vi "test_Generate State Information (JSON RCT).vi"(8 "error in":errorcluster) -> (0 "error out":errorcluster)   [LabVIEW 2020, in "Test_Routing Templates.lvlib"]
uses:
  Test_Routing Templates.lvlib
  Shared/Routing State.ctl
  Shared/Connection.ctl
  Routing Channel Templates/Abstract Routing Channel Template/Abstract Routing Channel Template.lvclass/Abstract Routing Channel Template.ctl
  Routing Channel Templates/JSON Routing Channel Template/JSON Routing Channel Template.lvclass
  C:/Users/mjacobso/Desktop/SCM/Routing-Faulting/Source/Routing and Faulting/Routing Templates/Routing Channel Templates/Abstract Routing Channel Template/Abstract Routing Channel Template.lvclass
  <vilib>/addons/_JKI Toolkits/Caraya/classes/Assert/Assert Equal Value_Variant.vi
  <vilib>/addons/_JKI Toolkits/Caraya/classes/Assert/Assert Error.vi
  <vilib>/addons/_JKI Toolkits/Caraya/classes/Test/Test.lvclass
  <vilib>/addons/_JKI Toolkits/Caraya/classes/Assert/Assert.lvclass
  Routing Channel Templates/Abstract Routing Channel Template/Abstract Routing Channel Template.lvclass
  Shared/Routing and Faulting Shared.lvlib
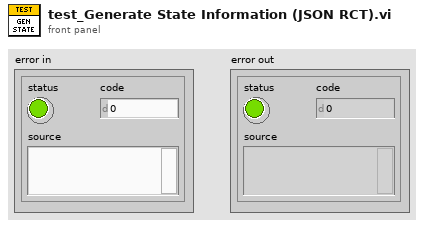
[diagram p1: front panel]
types:
  T1 = typedef "Routing and Faulting Shared.lvlib/Routing State.ctl" = cluster{"Name":string, "Description":string, "Value":i32, "Connection List":T2[]}
  T2 = typedef "Routing and Faulting Shared.lvlib/Connection.ctl" = cluster{"Module":string, "Source":string, "Destination":string}
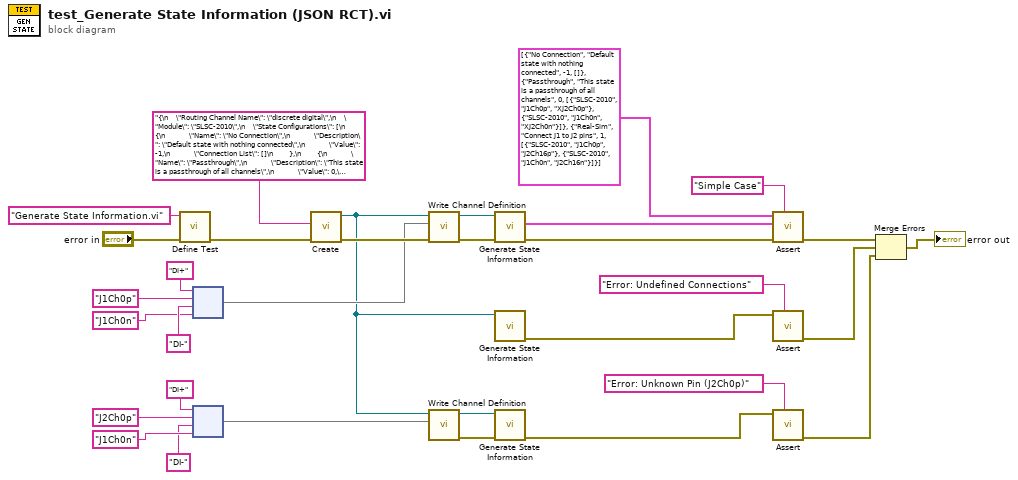
[diagram p0: block diagram]
diagram:
  n1 = call <vilib>:"Define Test.vi"("error in (no error)"="error in", "Label (VI Title)"="Generate State Information.vi") -> ("error out"=w29:errorcluster)  [unwired: 9 in]
  n2 = node("DI+", "J1Ch0p", "DI-", "J1Ch0n") -> (w22:map{string, string})
  n3 = node("DI+", "J2Ch0p", "DI-", "J1Ch0n") -> (w1:map{string, string})
  n4 = call "Create.vi"("error in (no error)"=w29, "JSON"="{\n    \"Routing Channel Name\": \"discrete digital\",\n    \"Module\": \"SLSC-2010\",\n    \"State Configurations\": [\n        {\n            \"Name\": \"No Connection\",\n            \"Description\": \"Default state with nothing connected\",\n            \"Value\": -1,\n            \"Connection List\": []\n        },\n        {\n            \"Name\": \"Passthrough\",\n            \"Description\": \"This state is a passthrough of all channels\",\n            \"Value\": 0,\n            \"Connection List\": [\n                {\n                    \"Channel\": \"DI+\",\n                    \"Connection Type\": \"Passthrough\"\n                },\n                {\n                    \"Channel\": \"DI-\",\n                    \"Connection Type\": \"Passthrough\"\n                }\n            ]\n        },\n        {\n            \"Name\": \"Real-Sim\",\n            \"Description\": \"Connect J1 to J2 pins\",\n            \"Value\": 1,\n            \"Connection List\": [\n                {\n                    \"Channel\": \"DI+\",\n                    \"Connection Type\": \"Real-Sim\"\n                },\n                {\n                    \"Channel\": \"DI-\",\n                    \"Connection Type\": \"Real-Sim\"\n                }\n            ]\n        }\n    ]\n}" ("text")) -> ("error out"=w27:errorcluster, "JSON Routing Channel Template out"=w8:refnum<class "JSON Routing Channel Template.lvclass">)  [unwired: 8 in]
  n5 = call "Write Channel Definition.vi"("error in (no error)"=w27, "Channel Definition"=w22, "Abstract Routing Channel Template in"=w8) -> ("error out"=w20:errorcluster, "Abstract Routing Channel Template out"=w19:refnum<class "JSON Routing Channel Template.lvclass">)  [unwired: 7 in]
  n6 = call "Write Channel Definition.vi"("Channel Definition"=w1, "Abstract Routing Channel Template in"=w8) -> ("error out"=w10:errorcluster, "Abstract Routing Channel Template out"=w9:refnum<class "JSON Routing Channel Template.lvclass">)  [unwired: 8 in]
  n7 = call-dynamic "Generate State Information.vi"("error in (no error)"=w20, "JSON RCT"=w19) -> ("error out"=w18:errorcluster, "State Configurations"=w17:T1[])  [unwired: 7 in, 1 out]
  n8 = call-dynamic "Generate State Information.vi"("JSON RCT"=w8) -> ("error out"=w12:errorcluster)  [unwired: 8 in, 2 out]
  n9 = call-dynamic "Generate State Information.vi"("error in (no error)"=w10, "JSON RCT"=w9) -> ("error out"=w7:errorcluster)  [unwired: 7 in, 2 out]
  n10 = call-poly <vilib>:"Assert.vi"("Label"="Simple Case", "error in (no error)"=w18, "Y"=w17, "X"=T1[] [{"Name"="No Connection", "Description"="Default state with nothing connected", "Value"=-1, "Connection List"=[]}, {"Name"="Passthrough", "Description"="This state is a passthrough of all channels", "Value"=0, "Connection List"=[{"Module"="SLSC-2010", "Source"="J1Ch0p", "Destination"="XJ2Ch0p"}, {"Module"="SLSC-2010", "Source"="J1Ch0n", "Destination"="XJ2Ch0n"}]}, {"Name"="Real-Sim", "Description"="Connect J1 to J2 pins", "Value"=1, "Connection List"=[{"Module"="SLSC-2010", "Source"="J1Ch0p", "Destination"="J2Ch16p"}, {"Module"="SLSC-2010", "Source"="J1Ch0n", "Destination"="J2Ch16n"}]}] ("State Configurations")) -> ("error out"=w30:errorcluster)  [unwired: 7 in]
  n11 = call-poly <vilib>:"Assert.vi"("Label"="Error: Undefined Connections", "Error?"=w12) -> ("error out"=w13:errorcluster)  [unwired: 9 in]
  n12 = call-poly <vilib>:"Assert.vi"("Label"="Error: Unknown Pin (J2Ch0p)", "Error?"=w7) -> ("error out"=w11:errorcluster)  [unwired: 9 in]
  n13 = Merge Errors(w30, w13, w11) -> (→"error out":errorcluster)
